vi "AC Source Type to AC Source lib type.vi"(11 "AWG type":T2) -> (3 "AWG lib type":T1)   [LabVIEW 2020]
doc: "Converts AC source type from actual project type definition to the type of the AWG library."
uses:
  external libraries/AWG/AWG Type.ctl
  external libraries/AWG/AWG.lvlib
  Type definitions/AC Source type.ctl
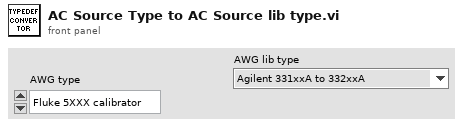
[diagram p1: front panel]
types:
  T1 = typedef "AWG.lvlib/AWG Type.ctl" = enum16{"Agilent 331xxA to 332xxA", "Agilent 335xxA to 336xxA", "Tektronix AFG3101C", "R&S HMF25xx", "CMI Clock Divider v2", "CMI Sync Unit V3", "dummy"}
  T2 = typedef "AC Source type.ctl" = enum16{"Fluke 5XXX calibrator", "Tektronix AFG3000 series", "dummy", "Agilent 331xxA to 332xxA", "Agilent 335xxA to 336xxA"}
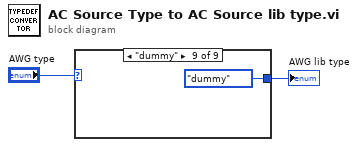
[diagram p0: block diagram]
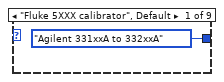
[diagram p2: hidden frame]
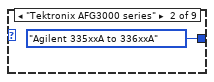
[diagram p3: hidden frame]
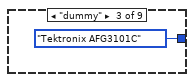
[diagram p4: hidden frame]
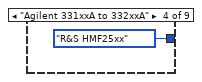
[diagram p5: hidden frame]
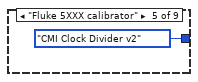
[diagram p6: hidden frame]
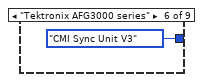
[diagram p7: hidden frame]
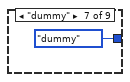
[diagram p8: hidden frame]
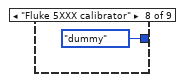
[diagram p9: hidden frame]
diagram:
  n1 = case shown="\"dummy\"" "AWG type" {
    tunnel: [AWG_Type."Agilent 331xxA to 332xxA" ("AWG type 2") AWG_Type."Agilent 335xxA to 336xxA" ("AWG type 2") AWG_Type."Tektronix AFG3101C" ("AWG type 2") AWG_Type."R&S HMF25xx" ("AWG type 2") AWG_Type."CMI Clock Divider v2" ("AWG type 2") AWG_Type."CMI Sync Unit V3" ("AWG type 2") AWG_Type."dummy" ("AWG type 2") AWG_Type."dummy" ("AWG type 2") AWG_Type."dummy" ("AWG type 2")] -> w1
    frame "Fluke 5XXX calibrator", Default {
    }
    frame "Tektronix AFG3000 series" {
    }
    frame "dummy" {
    }
    frame "Agilent 331xxA to 332xxA" {
    }
    frame "Fluke 5XXX calibrator" {
    }
    frame "Tektronix AFG3000 series" {
    }
    frame "dummy" {
    }
    frame "Fluke 5XXX calibrator" {
    }
    frame "dummy" {
    }
  }
  "AWG lib type" <- w1
